vi "GT Set Ext Io Bit.vi"(7 "value":u16, 8 "error in (no error)":errorcluster caption="错误输入（无错误）", 9 "index":i16, 10 "mdl":i16, 11 "cardNum":i16) -> (0 "error out":errorcluster caption="错误输出", 3 "function return":i16)   [LabVIEW 2014, in "gts.lvlib"]
doc: "GT_API GT_SetExtIoBit(short cardNum,short mdl,short index,unsigned short value);"
uses:
  gts.lvlib
  gts.dll
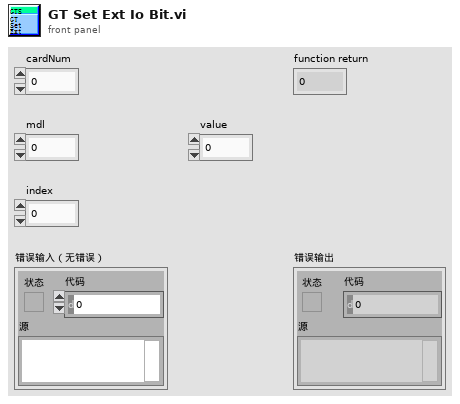
[diagram p1: front panel]
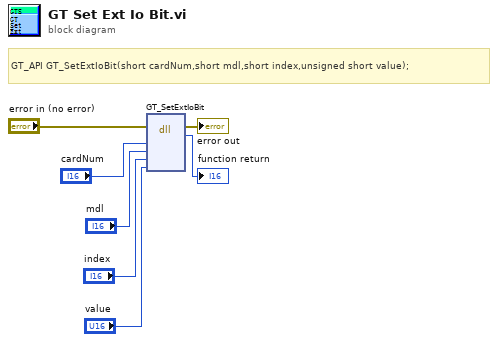
[diagram p0: block diagram]
diagram:
  # "GT_API GT_SetExtIoBit(short cardNum,short mdl,short index,unsigned short value);"
  n1 = dll-call lib="PTH2kabs D固高科技资料LABVIEWlabview 例程.多卡库-控制卡基本运动例程(labview)gts.*" fn="GT_SetExtIoBit"(error in="error in (no error)", "cardNum"="cardNum", "mdl"="mdl", "index"="index", "value"="value") -> (error out=→"error out":errorcluster, →"function return":i16)  [unwired: 6 in, 1 out]
